vi "Create Surface.vi"(6 "Draw Mode":T8(ring)=enum."Triangles", 7 "3D Surface Property":T1={"General Property"={"Plot Name"="", "Coordinate System"=enum."Cartesian", "Opacity"=0.0}, "Projection Property"={"Draw XY"=FALSE, "Draw YZ"=FALSE, "Draw XZ"=FALSE}, "Plot Property"={"Draw Surface"=FALSE, "Draw Mesh"=FALSE, "Draw Normal"=FALSE, "Color Ramp Cluster"={"Color Ramp Style"=enum."None", "Color Ramp Array"=[16711934, 393471, 57855, 4390754, 16449346, 16744722, 16711680], "Color Ramp Index"=[45, 91, 133, 175, 219, 255], "Interpolate?"=FALSE, "Logarithm?"=FALSE}, "Line Style"=enum."None", "Line Width"=0.0, "Line Color"=0, "Antialiasing"=FALSE}, "Surface Property"={"Color Mode"=enum."Flat Shading"}}, 8 "error in (no error)":errorcluster, 9 "Actual Transform In":T7, 10 "Plot Representation In":T4, 11 "Plot Object In":refnum<vi>) -> (0 "error out":errorcluster, 1 "Actual Transform Out":T7, 2 "Plot Representation Out":T4, 3 "Plot Object Out":refnum<vi>, 4 "Surface Object Out":refnum<vi>)   [LabVIEW 2017, in "3D Surface.lvclass"]
uses:
  <vilib>/Math Plots/3D Math Plots/3D Surface/3D Surface/3D Surface.lvclass
  <vilib>/Math Plots/3D Math Plots/3D Plot/3D Plot/Typedef/Actual Transform.ctl
  <vilib>/Math Plots/3D Math Plots/3D Plot/3D Plot/Typedef/Range Clusters.ctl
  <vilib>/Math Plots/3D Math Plots/3D Plot/3D Plot/Typedef/Plot Representation.ctl
  <vilib>/Math Plots/3D Math Plots/3D Plot/3D Plot/Typedef/Mesh Data.ctl
  <vilib>/Math Plots/3D Math Plots/3D Surface/3D Surface/Typedef/3D Surface Property.ctl
  <vilib>/Math Plots/3D Math Plots/3D Plot/3D Plot/Typedef/Color Ramp Cluster.ctl
  <vilib>/Math Plots/3D Math Plots/3D Plot/3D Plot/Typedef/Line Type.ctl
  <vilib>/picture/3D Picture Control/NI_3D Picture Control.lvlib
  <vilib>/Math Plots/3D Math Plots/3D Plot/3D Plot/3D Plot.lvclass
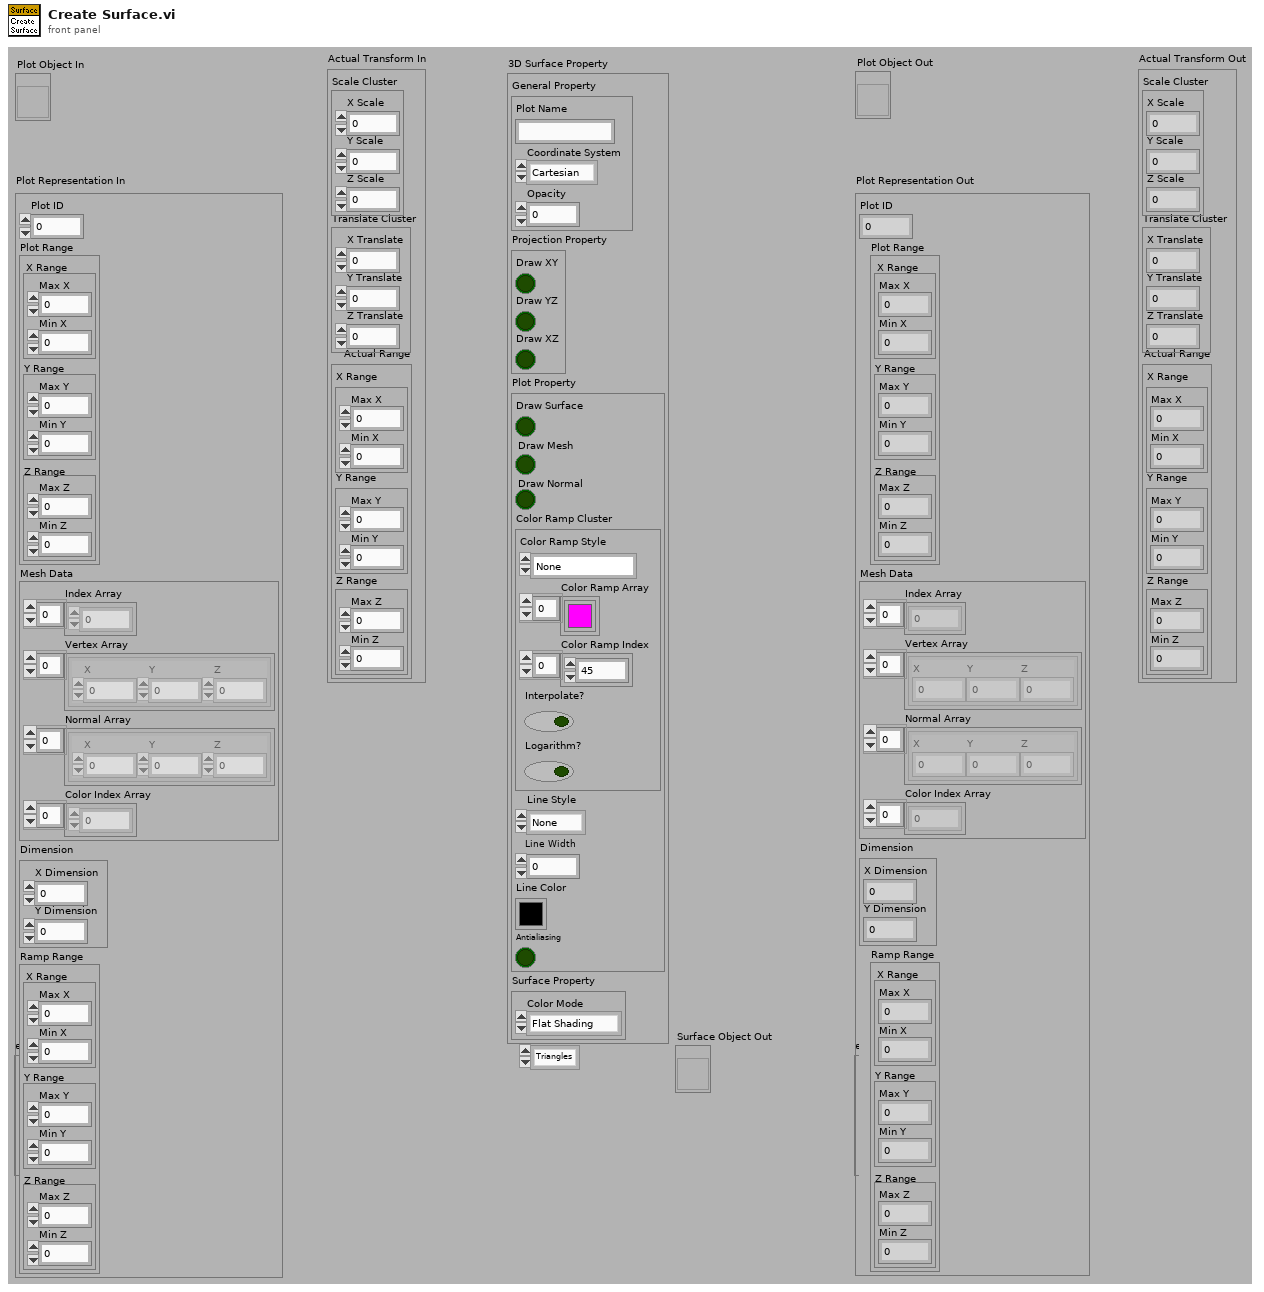
[diagram p1: front panel]
types:
  T1 = typedef "3D Surface.lvclass/3D Surface Property.ctl" = cluster{"General Property":cluster{"Plot Name":string, "Coordinate System":enum16{"Cartesian", "Cylindrical", "Spherical"}, "Opacity":sgl}, "Projection Property":cluster{"Draw XY":bool, "Draw YZ":bool, "Draw XZ":bool}, "Plot Property":cluster{"Draw Surface":bool, "Draw Mesh":bool, "Draw Normal":bool, "Color Ramp Cluster":T2, "Line Style":T3, "Line Width":sgl, "Line Color":u32, "Antialiasing":bool}, "Surface Property":cluster{"Color Mode":enum16{"Flat Shading", "Interpolated Shading"}}}
  T2 = typedef "3D Plot.lvclass/Color Ramp Cluster.ctl" = cluster{"Color Ramp Style":enum16{"None", "Shaded", "Color spectrum", "Grey scale", "Custom"}, "Color Ramp Array":u32[], "Color Ramp Index":i32[], "Interpolate?":bool, "Logarithm?":bool}
  T3 = typedef "3D Plot.lvclass/Line Type.ctl" = enum16{"None", "Solid", "Dash", "Dot", "Dash Dot"}
  T4 = typedef "3D Plot.lvclass/Plot Representation.ctl" = cluster{"Plot ID":i32, "Plot Range":T5, "Mesh Data":T6, "Dimension":cluster{"X Dimension":i32, "Y Dimension":i32}, "Ramp Range":T5}
  T5 = typedef "3D Plot.lvclass/Range Clusters.ctl" = cluster{"X Range":cluster{"Max X":sgl, "Min X":sgl}, "Y Range":cluster{"Max Y":sgl, "Min Y":sgl}, "Z Range":cluster{"Max Z":sgl, "Min Z":sgl}}
  T6 = typedef "3D Plot.lvclass/Mesh Data.ctl" = cluster{"Index Array":u32[], "Vertex Array":cluster{"X":sgl, "Y":sgl, "Z":sgl}[], "Normal Array":cluster{"X":sgl, "Y":sgl, "Z":sgl}[], "Color Index Array":i32[]}
  T7 = typedef "3D Plot.lvclass/Actual Transform.ctl" = cluster{"Scale Cluster":cluster{"X Scale":sgl, "Y Scale":sgl, "Z Scale":sgl}, "Translate Cluster":cluster{"X Translate":sgl, "Y Translate":sgl, "Z Translate":sgl}, "Actual Range":T5}
  T8 = enum16{"Points", "Lines", "Line Strip", "Line Loop", "Triangles", "Triangle Strip", "Triangle Fan", "Quads", "Quad Strip", "Polygon"}
  T9 = enum16{"Overall", "Per Primitive", "Per Vertex", "Binding Off"}
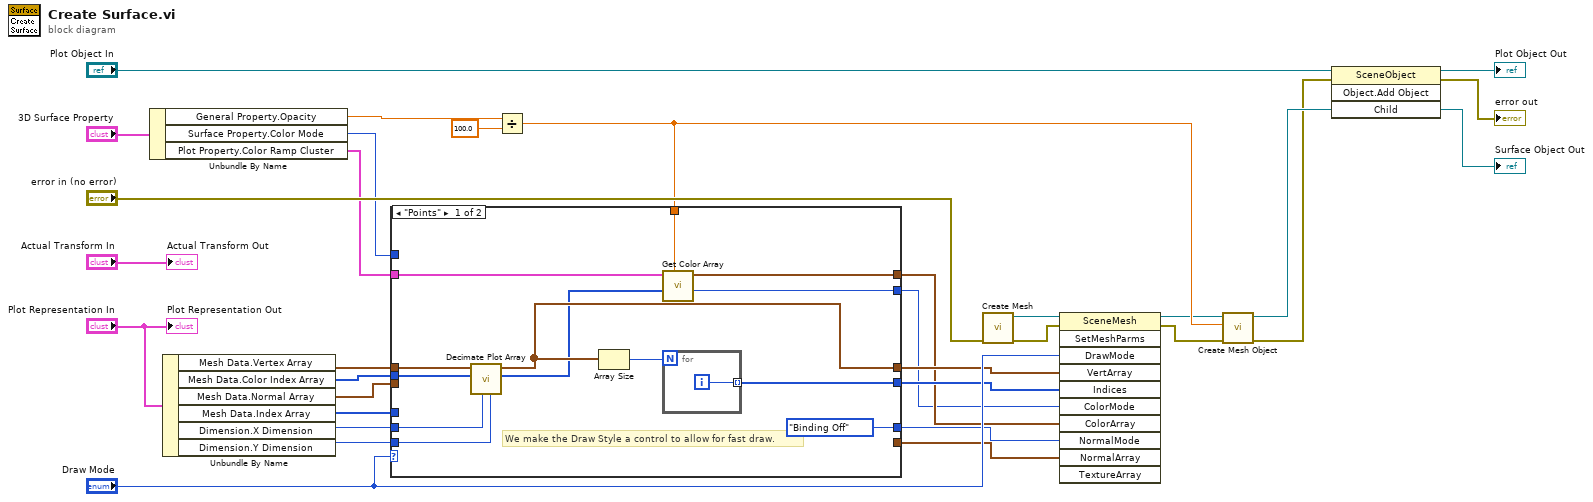
[diagram p0: block diagram]
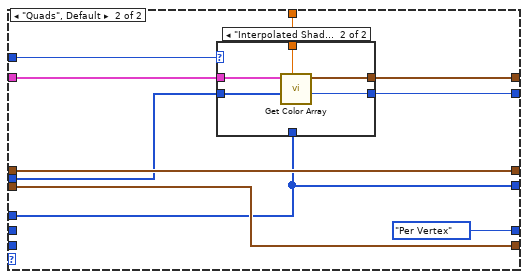
[diagram p2: hidden frame]
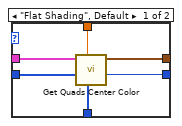
[diagram p3: hidden frame]
diagram:
  n1 = Unbundle By Name("3D Surface Property") -> ("General Property.Opacity"=w26:sgl, "Surface Property.Color Mode"=w12:enum16{"Flat Shading", "Interpolated Shading"}, "Plot Property.Color Ramp Cluster"=w10:T2)
  n2 = Unbundle By Name("Plot Representation In") -> ("Mesh Data.Vertex Array"=w18:cluster{"X":sgl, "Y":sgl, "Z":sgl}[], "Mesh Data.Color Index Array"=w11:i32[], "Mesh Data.Normal Array"=w17:cluster{"X":sgl, "Y":sgl, "Z":sgl}[], "Mesh Data.Index Array"=w9:u32[], "Dimension.X Dimension"=w16:i32, "Dimension.Y Dimension"=w15:i32)
  n3 = Divide(x=w26, y=sgl 100.0) -> (x/y=w8:sgl)
  n4 = case shown="\"Points\"" "Draw Mode" {
    tunnel: w18 -> [w44 w55]
    tunnel: [w41 w55] -> w23
    tunnel: [w35 w48] -> w25
    tunnel: w17 -> [_ w56]
    tunnel: [_ w56] -> w24
    tunnel: w16 -> [w43 _]
    tunnel: w15 -> [w42 _]
    tunnel: w10 -> [w34 w54]
    tunnel: w8 -> [w36 w53]
    tunnel: [w40 w52] -> w21
    tunnel: [w39 w51] -> w20
    tunnel: w12 -> [_ w50]
    tunnel: w11 -> [w38 w49]
    tunnel: w9 -> [_ w48]
    tunnel: [T9."Binding Off" ("Normal Binding Mode") T9."Per Vertex" ("Normal Binding Mode")] -> w7
    frame "Points" {
      # "We make the Draw Style a control to allow for fast draw."
      n5 = call <vilib>:"Decimate Plot Array.vi"("Y Dimension"=w42, "X Dimension"=w43, "Color Index Array In"=w38, "Vertex Array In"=w44) -> ("Color Index Array Out"=w37:i32[], "Vertex Array Out"=w41:cluster{"X":sgl, "Y":sgl, "Z":sgl}[])  [unwired: 1 in, 5 out]
      n6 = Array Size(array=w41) -> (size(s)=w45:i32)
      n7 = call <vilib>:"Get Color Array.vi"("Alpha"=w36, "Color Index Array"=w37, "Color Ramp Cluster"=w34) -> ("Color Binding Mode"=w39:T9, "Color Array"=w40:cluster{"R":sgl, "G":sgl, "B":sgl, "A":sgl}[])  [unwired: 3 in, 4 out]
      n8 = for {
        N: w45 -> [_]
        tunnel: [w46] -> w35 mode=indexing
        i -> [w46]
      }
    }
    frame "Quads", Default {
      n9 = case shown="\"Interpolated Shading\"" w50 {
        tunnel: w53 -> [w62 w64]
        tunnel: w54 -> [w57 w63]
        tunnel: [w59 w67] -> w52
        tunnel: [w58 w66] -> w51
        tunnel: w48 -> [w60 _]
        tunnel: w49 -> [w61 w65]
        frame "Flat Shading", Default {
          n10 = call <vilib>:"Get Quads Center Color.vi"("Index Array"=w60, "Alpha"=w62, "Color Index Array"=w61, "Color Ramp Cluster"=w57) -> ("Color Binding Mode"=w58:T9, "Color Array Out"=w59:cluster{"R":sgl, "G":sgl, "B":sgl, "A":sgl}[])  [unwired: 5 out]
        }
        frame "Interpolated Shading" {
          n11 = call <vilib>:"Get Color Array.vi"("Alpha"=w64, "Color Index Array"=w65, "Color Ramp Cluster"=w63) -> ("Color Binding Mode"=w66:T9, "Color Array"=w67:cluster{"R":sgl, "G":sgl, "B":sgl, "A":sgl}[])  [unwired: 3 in, 4 out]
        }
      }
    }
  }
  n12 = call <vilib>:"Create Mesh.vi"("error in (no error)"="error in (no error)") -> ("error out"=w4:errorcluster, "New Mesh Refnum"=w6:refnum<vi>)  [unwired: 9 out]
  n13 = invoke class="SceneMesh" method="SetMeshParms"(reference=w6, error in=w4, "DrawMode"="Draw Mode", "VertArray"=w23, "Indices"=w25, "ColorMode"=w20, "ColorArray"=w21, "NormalMode"=w7, "NormalArray"=w24) -> (reference out=w5:refnum<vi>, error out=w3:errorcluster)  [unwired: 2 in, 9 out]
  n14 = call <vilib>:"Create Mesh Object.vi"("error in (no error)"=w3, "Alpha"=w8, "Mesh Object In"=w5) -> ("error out"=w1:errorcluster, "Object Ref Out"=w2:refnum<vi>)  [unwired: 1 in, 6 out]
  n15 = invoke class="SceneObject" method="Object.Add Object"(reference="Plot Object In", error in=w1, "Child"=w2) -> (reference out=→"Plot Object Out":refnum<vi>, error out=→"error out":errorcluster, "Child"=→"Surface Object Out":refnum<vi>)  [unwired: 1 in, 1 out]
  "Actual Transform Out" <- "Actual Transform In"
  "Plot Representation Out" <- "Plot Representation In"
